vi "MAIN_RT.vi"() -> ()   [LabVIEW 2019]
uses:
  Modbus_class/ReadData.ctl
  Modbus_class/CMD REG.ctl
  Stand_class/Valve Mode.ctl
  <vilib>/Platform/TimedLoop/XDataNode/timing_clust.ctl
  <vilib>/Platform/TimedLoop/XDataNode/nitl_modes.ctl
  <vilib>/Platform/TimedLoop/XDataNode/wakeup.ctl
  Device_class/Device.lvclass/Device.ctl
  Proccess_class/Proccess.lvclass/Proccess.ctl
  Stand_class/Stand.lvclass/Stand.ctl
  AI_class/AI.lvclass/AI.ctl
  AnalogComparator_class/AnalogComparator.lvclass/AnalogComparator.ctl
  Modbus_class/ModbusSp.lvclass/ModbusSp.ctl
  PiecedLinearScale_class/Scale_PiecedLinear.lvclass/Scale_PiecedLinear.ctl
  Logger_class/Logger.lvclass/Logger.ctl
  dY_dX_Calculator/delayValue.lvclass/delayValue.ctl
  Valve_2DO_2DI_class/Valve_2DO_2DI.lvclass/Valve_2DO_2DI.ctl
  7973d5dc-5a66-4eb7-9f17-7206acf8e3d7.vi
  fa54bf54-d757-4f48-81c5-8c07d9776520.vi
  Device_class/ErrorToDb.vi/d458cff9-8e45-4544-91af-cfa5b3c8a69c.vi
  Proccess_class/GetNames.vi
  Modbus_class/ReadMbDat.vi
  AI_class/SetRaw.vi
  Device_class/Modbusd cmd to db.vi
  Modbus_class/WriteMbDat.vi
  Stand_class/Prepare Data Modbus STS.vi
  AI_class/Get_Values.vi
  dY_dX_Calculator/Update.vi
  Stand_class/Handle dP dT.vi/d0b32f7e-a2eb-4dff-9ec3-f7480154de2a.vi
  dY_dX_Calculator/Config.vi
  Stand_class/private/ExecuteStep.vi
  Stand_class/Handle Drain.vi
  Stand_class/Handle Mode.vi/285b69a7-cd4c-45dd-8dd6-80699296fb4f.vi
  Stand_class/calc sp go up.vi
  Stand_class/Handle 44_1_2.vi
  Device_class/GetFPGA.vi
  Stand_class/Valve State Mode.vi
  Modbus_class/ConvertRegToReadData.vi
  Modbus_class/Clear CMD Reg.vi
  PiecedLinearScale_class/RawToScaled.vi
  subvis/Average.vi
  AI_class/HandleRanges.vi
  AI_class/private/WriteToDb.vi
  Modbus_class/ConvertWriteDataToReg.vi
  AnalogComparator_class/GetStatus.vi
  Stand_class/Nitro and Dut.vi
  Stand_class/Set Hi Press.vi
  Stand_class/Invert Direction.vi
  Stand_class/private/ExecuteStep.vi/d900ba76-673b-43eb-b747-4a40eb4a2de0.vi
  Stand_class/calc sp go up.vi/c91f4351-afbf-4a48-b204-0d489dec29b1.vi
  Stand_class/calc sp go up.vi/50fb84da-4633-4161-b856-f10d1b653a37.vi
  Valve_2DO_2DI_class/GetState.vi
  Valve_2DO_2DI_class/Open.vi
  Stand_class/Handle 44_1_2.vi/53daa488-cb92-467d-8939-09c81072894d.vi
  Stand_class/Handle 44_1_2.vi/27880750-5bda-4793-8800-8ef0418d5d30.vi
  Stand_class/Valve State Mode.vi/810e184e-eeb6-4027-a8ae-1422f3ce3d45.vi
  Stand_class/Valve State Mode.vi/57bd4a65-f3dc-44f5-8d68-677c2a197570.vi
  Stand_class/Valve State Mode.vi/03b2f9e4-fceb-4725-9b90-3fd10082a088.vi
  Stand_class/Valve State Mode.vi/3d0d09bd-48e8-482f-b1e2-a36b2bb65234.vi
  Stand_class/Valve State Mode.vi/33d3f26a-dc4a-4f56-bf0a-61d04c5d7434.vi
  Stand_class/Valve State Mode.vi/52af9d47-24d1-4057-80bf-8d93bfb3d17d.vi
  Stand_class/Valve State Mode.vi/094228cb-a119-423c-9af8-5a16f059a318.vi
  Stand_class/Valve State Mode.vi/bf5ad1e6-a0ae-4579-ad74-ca8f304cb7cf.vi
  Stand_class/Valve State Mode.vi/eb4d2b76-f0f0-4e1d-bda0-609c5f37b4e7.vi
  Modbus Data Type Conversation/U16 Array TO SGL Array.vi
  AnalogComparator_class/SetValue.vi
  Logger_class/Enqueue Signal.vi
  Modbus Data Type Conversation/SGL Array to U16 Array.vi
  Stand_class/Haskel Fast Forward.vi
  Stand_class/Set Hi Press.vi/29706e3b-acf2-4be0-8e3a-420f003c1de5.vi
  Modbus Data Type Conversation/SGL to U16.vi
  subvis/FastForward.vi
  Stand_class/Get U max Haskel.vi
  Stand_class/Get Accuracy.vi
  Stand_class/Stand.lvclass
  C:/Users/ANENKOV_V1/Desktop/SRC_H400/src/Proccess_class/Proccess.lvclass
  C:/Users/ANENKOV_V1/Desktop/SRC_H400/src/Device_class/Device.lvclass
  Device_class/Device.lvclass
  AI_class/AI.lvclass
  Valve_2DO_2DI_class/Valve_2DO_2DI.lvclass
  <vilib>/Utility/error.llb/Error Cluster From Error Code.vi
  Stand_class/Const All Valve.vi
  Logger_class/WriteEvent.vi
  simple_udp/Global - Pressure Data.vi
  <vilib>/gmath/interp.llb/Interpolate 1D.vi
  AnalogComparator_class/SendToDb.vi
  Stand_class/Handle MB Commands.vi
  Modbus_class/STS Cluster to REG.vi
  Modbus_class/Conection List.vi
  Global/Global Constant.vi
  Stand_class/private/Filling.vi
  Stand_class/private/Init Step.vi
  Stand_class/Set Backpressure.vi
  Stand_class/PreLoading.vi
  <vilib>/addons/_JKI.lib/FPGA_Basic_Components/Counter JKI_FPGA.vi
  <vilib>/addons/_JKI.lib/FPGA_Basic_Components/Counter_32bit JKI_FPGA.vi
  NeedleValve_class/Do.vi
  Stand_class/private/Check Range Hi Press.vi
  Stand_class/Down Pressure.vi
  Stand_class/Set Ziro.vi
  Stand_class/Check Step is Done.vi
  PM_Group_class/All Stop.vi
  <vilib>/ErrorRing/Error Ring.xnode
  <vilib>/platform/TimedLoop/XDataNode/XDataNode.xnode
  Logger_class/Logger.lvclass
  FPGA_API_class/FPGA API.lvclass
  <vilib>/NI/Modbus Library/API/Slave/Modbus Slave.lvclass
  <vilib>/Platform/TimedLoop/XDataNode/XDNodeRunTimeDep.lvlib
  Libs/RT_Shared_Variables.lvlib
  <vilib>/NI/AMC/AMC.lvlib
  SV_Puplisher_class/SV_Publisher.lvclass
  Proccess_class/Proccess.lvclass
  Modbus_class/ModbusSp.lvclass
panel:
  in  "set":bool
  in  "Valve DIR":T1
  out "mb cmd log":string
  out "dt ms handle mode":u32
  out "dt ms (dp/dt)":u32
  in  "CMD REG":T2
  out "Data Read":T3
  out "dt":i64
  out "String":string
  out "dt all":u32
  out "error hmi":errorcluster
  out "dt handle alarms":u32
  out "dt dev":u32
  out "dt handle cmd":u32
  out "dt public sv":u32
  out "dt fpga":u32
  out "Error NV":errorcluster
  out "Error SV Public":errorcluster
  out "error main":errorcluster
  in  "stop":bool
  out "Iteration Duration":i64
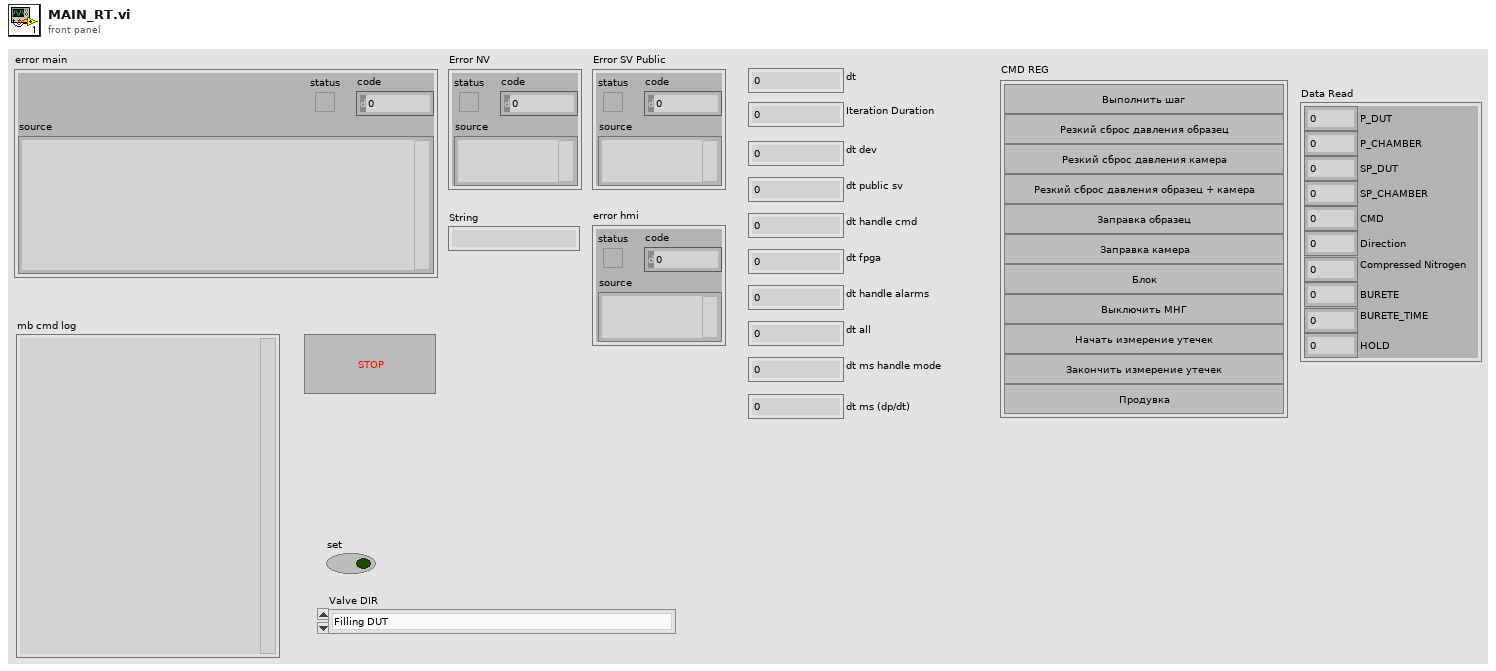
[diagram p1: front panel]
types:
  T1 = typedef "Valve Mode.ctl" = enum16{"Filling DUT", "Filling Chamber", "Pump Pressure DUT", "Pump Pressure Chamber", "Haskel Pressure DUT", "Haskel Pressure Chamber", "Slow Release DUT", "Slow Release Chamber", "Fast Release DUT", "Fast Release Chamber", "Fast Release DUT and Chamber", "Leak Pressure DUT", "Leak Pressure Chamber", "Back Pressure DUT", "Back Pressure Chamber", "Fully Closed", "Drain", "Block DUT", "Block Chamber"}
  T2 = typedef "CMD REG.ctl" = cluster{"EXECUTE_SP":bool, "ALARM_PRESS_DOWN_DUT":bool, "ALARM_PRESS_DOWN_CHAMBER":bool, "ALARM_PRESS_DOWN_DUT_CHAMBER":bool, "FILING_DUT":bool, "FILING_CHAMBER":bool, "BLOCK":bool, "PUMP_STATION_OFF":bool, "Leak start":bool, "Leak stop":bool, "Drain":bool}
  T3 = typedef "ModbusSp.lvclass/ReadData.ctl" = cluster{"P_DUT":sgl, "P_CHAMBER":sgl, "SP_DUT":sgl, "SP_CHAMBER":sgl, "CMD":u16, "Direction":u16, "Compressed Nitrogen":u16, "BURETE":u16, "BURETE_TIME":u16, "HOLD":u16}
  T4 = typedef "XDNodeRunTimeDep.lvlib/timing_clust.ctl" = cluster{"Expected End [f-1]":u64, "Actual End [f-1]":u64, "Finished Late? [f-1]":bool, "Expected End [i-1]":u64, "Actual End [i-1]":u64, "Finished Late? [i-1]":bool, "Expected Start [i]":u64, "Actual Start [i]":u64, "Expected Start [f]":u64, "Actual Start [f]":u64, "Source Name":string, "Structure Name":string, "Period":i64, "Deadline":i64, "Offset":i64, "Start":i64, "Priority":i32, "Timeout":i32, "Mode":T5, "Wakeup Reason":T6, "Error":errorcluster, "Source Type":string, "Secondary Source Type":string, "Global End Time":u64, "Global Start Time":u64, "Frame Duration":u64, "Iteration Duration":u64, "Assigned CPU":i32, "I/O Scan Engine Mode":u32}
  T5 = typedef "XDNodeRunTimeDep.lvlib/nitl_modes.ctl" = enum32{"No Change", "Process missed periods, maintain original phase", "Discard missed periods, maintain original phase", "Process missed periods, ignore original phase", "Discard missed periods, ignore original phase"}
  T6 = typedef "XDNodeRunTimeDep.lvlib/wakeup.ctl" = enum32{"Normal", "Aborted", "Asynchronous wakeup", "Timing source error", "Timed loop error", "Timeout"}
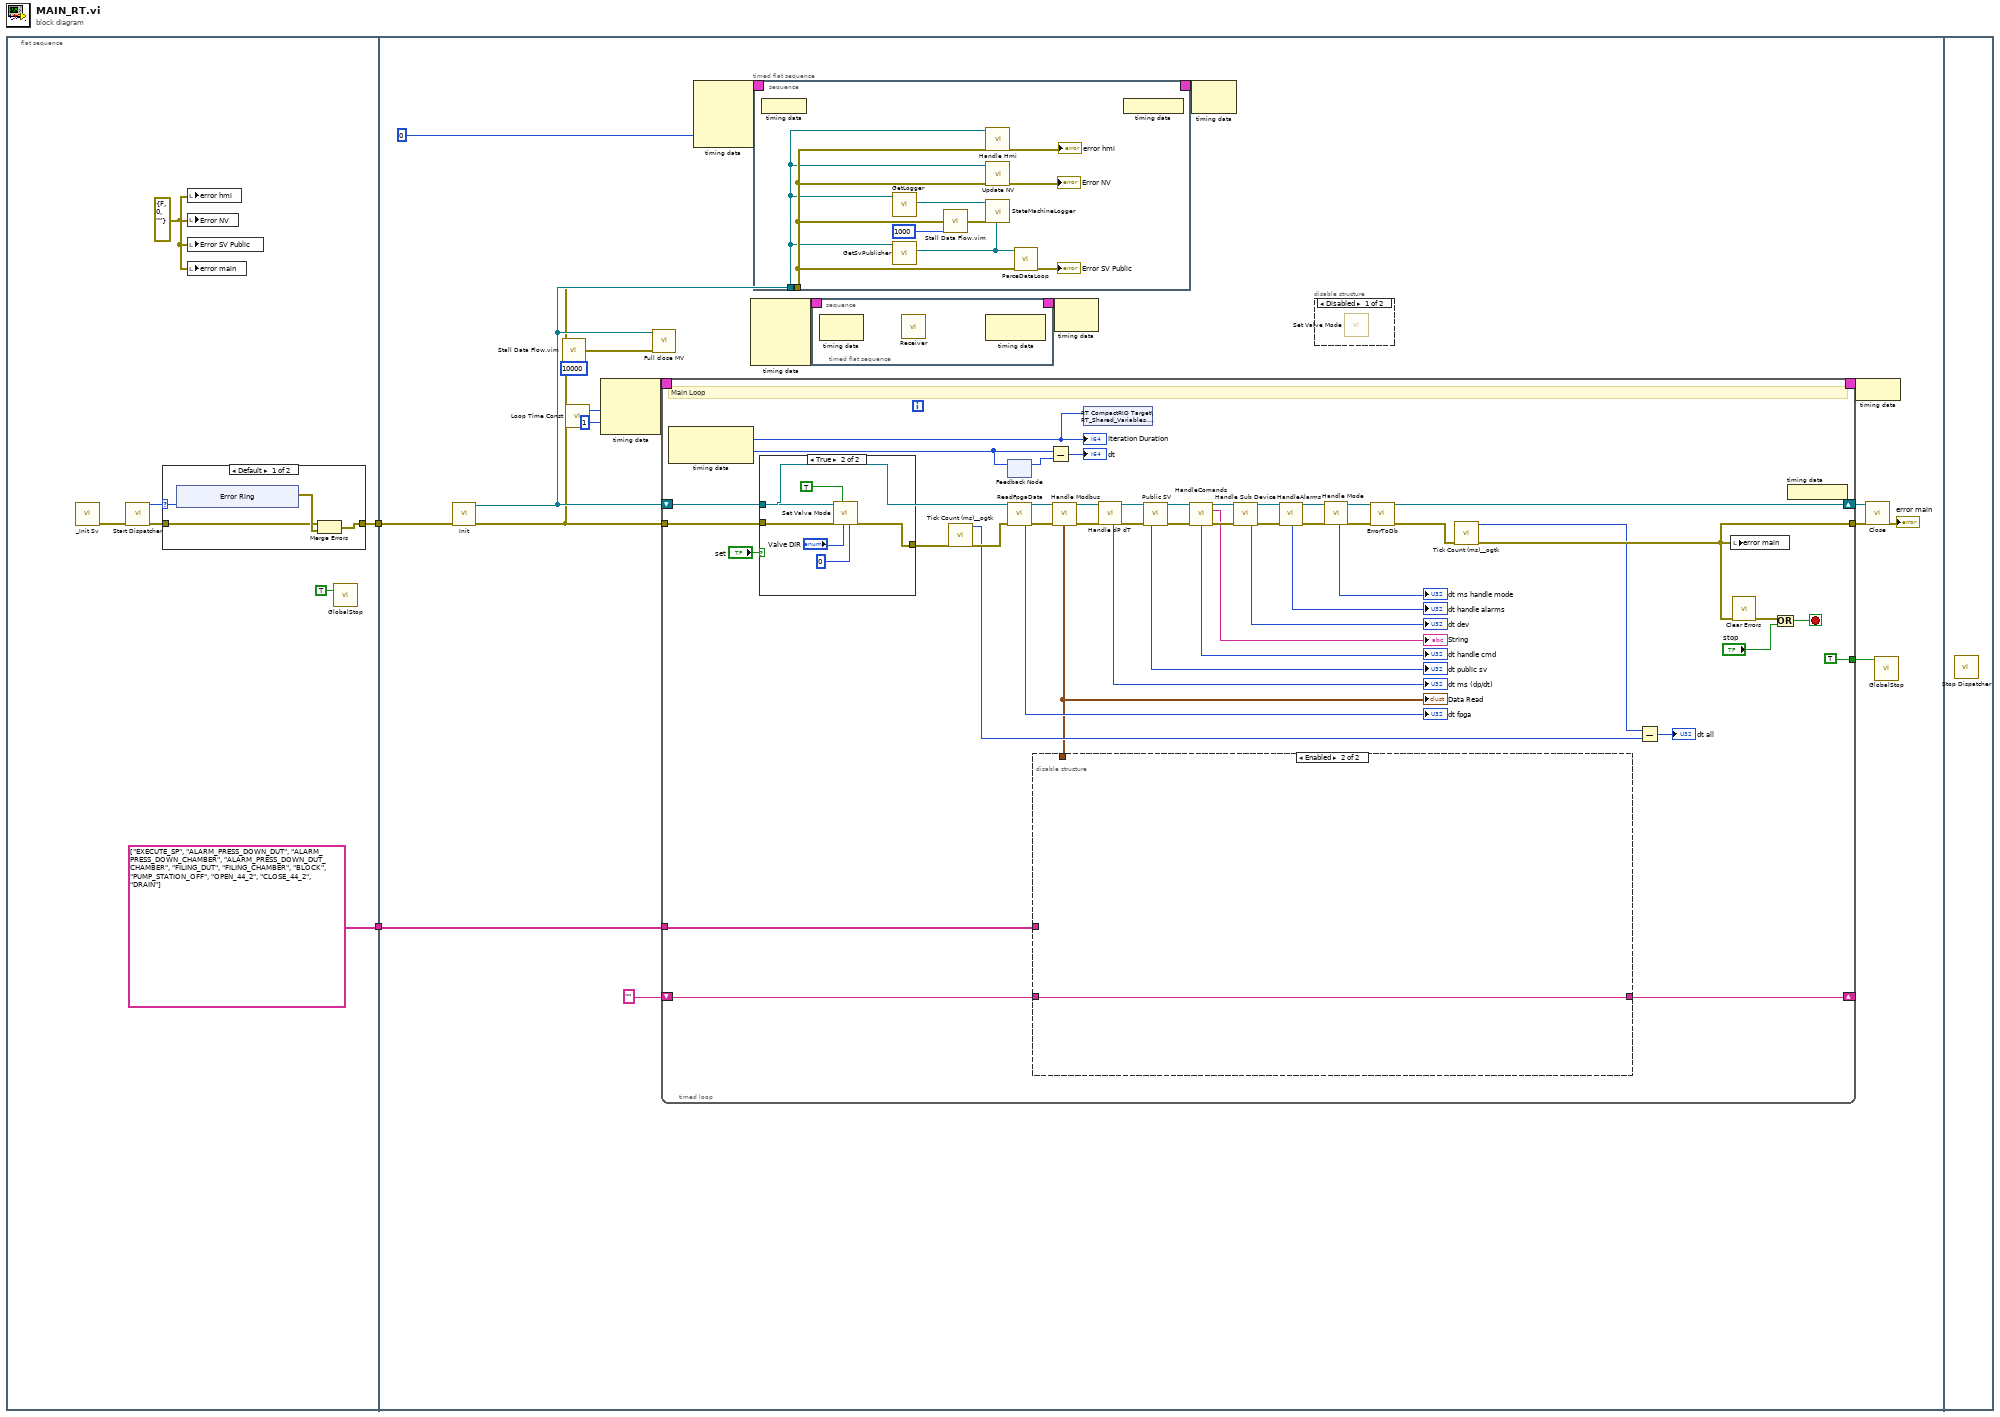
[diagram p0: block diagram]
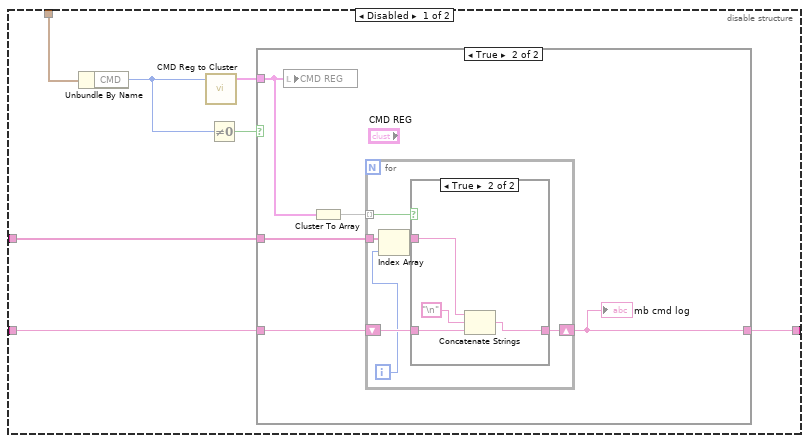
[diagram p5: hidden frame]
diagram:
  n1 = flat-sequence {
    tunnel: [w7] -> w2
    tunnel: [string[] ["EXECUTE_SP", "ALARM_PRESS_DOWN_DUT", "ALARM_PRESS_DOWN_CHAMBER", "ALARM_PRESS_DOWN_DUT_CHAMBER", "FILING_DUT", "FILING_CHAMBER", "BLOCK", "PUMP_STATION_OFF", "OPEN_44_2", "CLOSE_44_2", "DRAIN"] ("Array")] -> w1
    tunnel: w2 -> [w36]
    tunnel: w1 -> [w25]
    frame #0 {
      w4 = errorcluster {"status"=FALSE, "code"=0, "source"=""} ("error mb")
      n2 = call "_Init Sv.vi"() -> ("error out"=w9:errorcluster)  [unwired: 15 in]
      n3 = call <vilib>:"Start Dispatcher.vi"("error in"=w9) -> ("UDP port used"=w8:u16, "error out"=w6:errorcluster)  [unwired: 12 in, 1 out]
      n4 = case shown="Default" w8 {
        selector: w8 -> [w10 _]
        tunnel: [w13 w21] -> w7
        tunnel: w6 -> [w11 w21]
        frame Default {
          n5 = xnode "Error Ring"("parameter 0"=w10) -> ("error out"=w12:errorcluster)
          n6 = Merge Errors(w11, w12) -> (w13:errorcluster)
        }
        frame 54321 {
        }
      }
      n7 = local write "error hmi"(w4) -> ()
      n8 = local write "Error NV"(w4) -> ()
      n9 = local write "Error SV Public"(w4) -> ()
      n10 = local write "error main"(w4) -> ()
      n11 = call "GlobalStop.vi"("Reset"=TRUE) -> ()  [unwired: 14 in, 1 out]
    }
    frame #1 {
      n12 = call "Init.vi"("error in (no error)"=w36) -> ("error out"=w28:errorcluster, "Stand out"=w29:refnum<class "Stand.lvclass">)  [unwired: 9 in]
      n13 = call "Stall Data Flow.vim"("value in"=w28, "milliseconds to wait"=u32 10000) -> ("value out"=w27:errorcluster)  [unwired: 1 out]
      n14 = call "Loop Time Const.vi"() -> ("loop time ms"=w34:i64)  [unwired: 3 in]
      n15 = node-c288(w34, 1 ("Processor")) -> (w41:T4)  [unwired: 1 in]
      n16 = call "Full close MV.vi"("error in (no error)"=w27, "Stand in"=w29) -> ()  [unwired: 9 in, 1 out]
      n17 = timed-loop {
        timing: w41 -> [_]
        timing-out: [_] -> w40
        shift-right: [w95] -> w39
        shift-left: w29 -> [w60]
        tunnel: w28 -> [w62]
        tunnel: [w90] -> w38
        tunnel: [TRUE ("Reset")] -> w35
        tunnel: w25 -> [w66]
        shift-right: [w64] -> _
        shift-left: "" -> [w65]
        stop <- w97 stop-if-true
        # "Main Loop"
        n18 = node-c288() -> (w63:i64, w71:i64)  [unwired: 1 in]
        "Iteration Duration" <- w63
        n19 = case shown="True" "set" {
          tunnel: w62 -> [w106 w111]
          tunnel: [w106 w108] -> w61
          tunnel: w60 -> [_ w107]
          frame False {
          }
          frame True {
            n20 = call "Set Valve Mode.vi"("time after close"=u32 0, "Valve DIR"="Valve DIR", "init"=TRUE, "error in (no error)"=w111, "Stand in"=w107) -> ("error out"=w108:errorcluster)  [unwired: 5 in, 1 out]
          }
        }
        n21 = call <userlib>:"Tick Count (ms)__ogtk.vi"("error in (no error)"=w61) -> ("error out"=w92:errorcluster, "millisecond timer value"=w87:u32)  [unwired: 9 in]
        n22 = feedback #1() -> (w72:i64)  [unwired: 1 in]
        n23 = feedback-in #1(w71) -> ()
        n24 = call "ReadFpgaData.vi"("Stand"=w60, "error in (no error)"=w92) -> ("Stand out"=w84:refnum<class "Stand.lvclass">, "dt"=→"dt fpga":u32, "error out"=w83:errorcluster)  [unwired: 11 in]
        n25 = Subtract(x=w71, y=w72) -> (x-y=→"dt":i64)
        n26 = call "Handle Modbus.vi"("reference in"=w84, "error in (no error)"=w83) -> ("reference out"=w81:refnum<class "Stand.lvclass">, "Data Read"=w67:T3, "error out"=w82:errorcluster)  [unwired: 11 in]
        "Data Read" <- w67
        n27 = disable-structure shown="Enabled" {
          disable-tunnel: w67 -> [w119 _]
          disable-tunnel: w66 -> [w115 _]
          disable-tunnel: w65 -> [w114 w137]
          disable-tunnel: [w113 w137] -> w64
          frame Disabled {
            n28 = Unbundle By Name(w119) -> ("CMD"=w117:u16)
            n29 = call "CMD Reg to Cluster.vi"("CMD Reg"=w117) -> ("CMD REG"=w116:T2)  [unwired: 14 in]
            n30 = Not Equal To 0?(x=w117) -> (x != 0?=w118:bool)
            n31 = case shown="True" w118 {
              tunnel: w116 -> [_ w125]
              tunnel: w115 -> [_ w123]
              tunnel: w114 -> [w120 w122]
              tunnel: [w120 w121] -> w113
              frame False {
              }
              frame True {
                n32 = local write "CMD REG"(w125) -> ()
                n33 = Cluster To Array(cluster=w125) -> (array=w124:bool[])
                n34 = for {
                  tunnel: w124 -> [w131] mode=indexing
                  tunnel: w123 -> [w130]
                  shift-right: [w128] -> w121
                  shift-left: w122 -> [w129]
                  i -> [w126]
                  n35 = Index Array(array=w130, index=w126) -> (element=w127:string)
                  n36 = case shown="True" w131 {
                    tunnel: w127 -> [_ w135]
                    tunnel: w129 -> [w132 w136]
                    tunnel: [w132 w133] -> w128
                    frame False {
                    }
                    frame True {
                      n37 = Concatenate Strings(w135, "\n", w136) -> (w133:string)
                    }
                  }
                }
                "mb cmd log" <- w121
              }
            }
          }
          frame Enabled {
          }
        }
        n38 = shared-variable "RT CompactRIO Target\\RT_Shared_Variables.lvlib\\duration"(w63) -> ()  [unwired: 1 in, 1 out]
        n39 = call "Handle dP dT.vi"("error in (no error)"=w82, "Stand in"=w81) -> ("error out"=w86:errorcluster, "Stand out"=w85:refnum<class "Stand.lvclass">, "dt ms"=→"dt ms (dp/dt)":u32)  [unwired: 7 in]
        n40 = call "Public SV.vi"("reference in"=w85, "error in (no error)"=w86) -> ("reference out"=w96:refnum<class "Stand.lvclass">, "dt public sv"=→"dt public sv":u32, "error out"=w105:errorcluster)  [unwired: 11 in]
        n41 = call "HandleComands.vi"("Stand in"=w96, "error in (no error)"=w105) -> ("Stand out"=w79:refnum<class "Stand.lvclass">, "String"=→"String":string, "dt handle cmd"=→"dt handle cmd":u32, "error out"=w80:errorcluster)  [unwired: 10 in]
        n42 = call "Handle Sub Device.vi"("Stand in"=w79, "error in (no error)"=w80) -> ("Stand out"=w93:refnum<class "Stand.lvclass">, "dt PMG"=→"dt dev":u32, "error out"=w94:errorcluster)  [unwired: 11 in]
        n43 = call "HandleAlarms.vi"("Stand in"=w93, "error in (no error)"=w94) -> ("Stand out"=w76:refnum<class "Stand.lvclass">, "dt handle alarms"=→"dt handle alarms":u32, "error out"=w75:errorcluster)  [unwired: 11 in]
        n44 = call "Handle Mode.vi"("error in (no error)"=w75, "Stand in"=w76) -> ("error out"=w74:errorcluster, "Stand out"=w73:refnum<class "Stand.lvclass">, "dt ms handle mode"=→"dt ms handle mode":u32)  [unwired: 7 in]
        n45 = call "ErrorToDb.vi"("reference in"=w73, "error in (no error)"=w74) -> ("reference out"=w95:refnum<class "Stand.lvclass">, "error out"=w91:errorcluster)  [unwired: 12 in]
        n46 = call <userlib>:"Tick Count (ms)__ogtk.vi"("error in (no error)"=w91) -> ("error out"=w90:errorcluster, "millisecond timer value"=w89:u32)  [unwired: 9 in]
        n47 = Subtract(x=w89, y=w87) -> (x-y=→"dt all":u32)
        n48 = local write "error main"(w90) -> ()
        n49 = call <vilib>:"Clear Errors.vi"("error in (no error)"=w90) -> ("error out"=w77:errorcluster)  [unwired: 5 in, 1 out]
        n50 = Or(x=w77, y="stop") -> (x .or. y?=w97:bool)
        n51 = node-c288() -> ()  [unwired: 1 out]
      }
      n52 = node-c288(0 ("Processor")) -> (w33:T4)  [unwired: 3 in]
      n53 = node-c288() -> (w23:T4)  [unwired: 4 in]
      n54 = timed-sequence "Timed Sequence" {
        timing: w33 -> [_]
        timing-out: [_] -> w32
        tunnel: w29 -> [w47]
        tunnel: w28 -> [w46]
        n55 = timed-flat-sequence {
          tunnel: w47 -> [w49]
          tunnel: w46 -> [w50]
          n56 = node-c288() -> ()  [unwired: 1 in]
          n57 = call "GetLogger.vi"("Proccess in"=w49) -> ("Logger"=w54:refnum<class "Logger.lvclass">)  [unwired: 10 in]
          n58 = call "GetSvPublisher.vi"("Device in"=w49) -> ("SV_Publisher.lvclass"=w56:refnum<class "SV_Publisher.lvclass">)  [unwired: 10 in]
          n59 = call "Stall Data Flow.vim"("value in"=w50, "milliseconds to wait"=u32 1000) -> ("value out"=w52:errorcluster)  [unwired: 1 out]
          n60 = call "Handle Hmi.vi"("error in (no error)"=w50, "Stand in"=w49) -> ("error out"=→"error hmi":errorcluster)  [unwired: 8 in, 1 out]
          n61 = call "Update NV.vi"("error in (no error)"=w50, "Stand in"=w49) -> ("error out"=→"Error NV":errorcluster)  [unwired: 9 in]
          n62 = call-dynamic "StateMachineLogger.vi"("reference in"=w54, "error in (no error)"=w52, "SV_Publisher in"=w56) -> ()  [unwired: 17 in]
          n63 = call "ParceDataLoop.vi"("error in (no error)"=w50, "SV_Publisher in"=w56) -> ("error out"=→"Error SV Public":errorcluster)  [unwired: 9 in]
          n64 = node-c288() -> ()  [unwired: 1 out]
        }
      }
      n65 = timed-sequence {
        timing: w23 -> [_]
        timing-out: [_] -> w22
        n66 = timed-flat-sequence {
          n67 = node-c288() -> ()  [unwired: 1 in, 1 out]
          n68 = call "Receiver.vi"() -> ()  [unwired: 16 in]
          n69 = node-c288() -> ()  [unwired: 1 in, 1 out]
        }
      }
      n70 = node-c288(w22) -> ()  [unwired: 1 out]
      n71 = node-c288(w32) -> ()  [unwired: 1 out]
      n72 = disable-structure shown="Disabled" {
        frame Disabled {
          n73 = call "Set Valve Mode.vi"() -> ()  [unwired: 10 in, 2 out]
        }
        frame Enabled {
        }
      }
      n74 = node-c288(w40) -> ()
      n75 = call "Close.vi"("error in (no error)"=w38, "Stand in"=w39) -> ("error out"=→"error main":errorcluster)  [unwired: 9 in]
      n76 = call "GlobalStop.vi"("Set"=w35) -> ()  [unwired: 14 in, 1 out]
    }
    frame #2 {
      n77 = call <vilib>:"Stop Dispatcher.vi"() -> ()  [unwired: 15 in, 1 out]
    }
  }
